vi "System Display Settings.vi"(0 "VISA resource name":refnum<visa-resource-name>, 1 "Result Mode (0:Mode A)":i32(ring) items=["Mode A", "Mode B"], 5 "Enable Sound (1:On)":i32(ring)=1 items=["Off", "On"], 7 "LCD Display Mode (1:On)":i32(ring)=1 items=["Off", "On"], 9 "Uncal Display Mode (1:On)":i32(ring)=1 items=["Off", "On"], 11 "error in (no error)":errorcluster, 12 "Display Title (1:Show Title Display)":i32(ring)=1 items=["No Title Display", "Show Title Display", "Erase Warmup Message"], 13 "Title":string) -> (4 "VISA resource name out":refnum<visa-resource-name>, 15 "error out":errorcluster)   [LabVIEW 2020, in "Anritsu Signal Analyzer Series.lvlib"]
doc: "Sets the system or display settings for sound, LCD, Uncal, and Result mode settings."
uses:
  Anritsu Signal Analyzer Series.lvlib
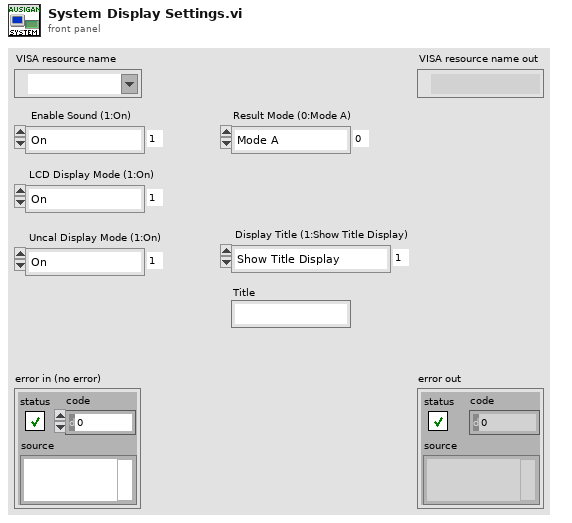
[diagram p1: front panel]
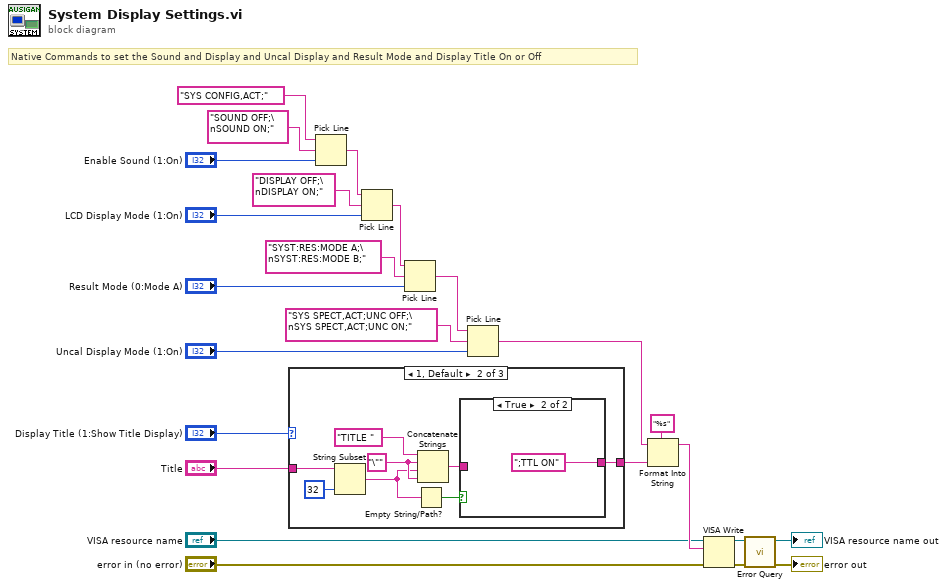
[diagram p0: block diagram]
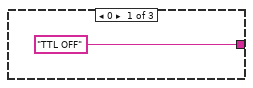
[diagram p2: hidden frame]
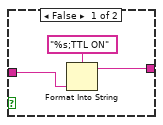
[diagram p3: hidden frame]
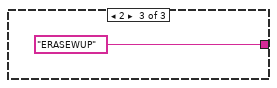
[diagram p4: hidden frame]
diagram:
  # "Native Commands to set the Sound and Display and Uncal Display and Result Mode and Display Title On or Off"
  n1 = case shown="1, Default" "Display Title (1:Show Title Display)" {
    tunnel: ["TTL OFF" ("_CommandSet") w29 "ERASEWUP" ("_CommandSet")] -> w12
    tunnel: "Title" -> [_ w28 _]
    frame 0 {
    }
    frame 1, Default {
      w33 = "\"" ("string")
      n2 = String Subset(string=w28, length (rest)=32 ("length (rest)")) -> (substring=w27:string)  [unwired: 1 in]
      n3 = Empty String/Path?(string/path=w27) -> (empty?=w26:bool)
      n4 = Concatenate Strings("TITLE " ("_CommandSet"), w33, w27, w33) -> (w30:string)
      n5 = case shown="True" w26 {
        tunnel: w30 -> [w35 _]
        tunnel: [w34 ";TTL ON" ("形式文字列")] -> w29
        frame False {
          n6 = Format Into String(format string="%s;TTL ON" ("形式文字列"), w35) -> (resulting string=w34:string)  [unwired: 2 in, 1 out]
        }
        frame True {
        }
      }
    }
    frame 2 {
    }
  }
  n7 = Pick Line(string ("")="SYS CONFIG,ACT;" ("_Case1"), multi-line string="SOUND OFF;\nSOUND ON;" ("_Case1"), line index="Enable Sound (1:On)") -> (output string=w14:string)
  n8 = Pick Line(string ("")=w14, multi-line string="DISPLAY OFF;\nDISPLAY ON;" ("_Case1"), line index="LCD Display Mode (1:On)") -> (output string=w8:string)
  n9 = Pick Line(string ("")=w8, multi-line string="SYST:RES:MODE A;\nSYST:RES:MODE B;" ("_Case1"), line index="Result Mode (0:Mode A)") -> (output string=w1:string)
  n10 = Pick Line(string ("")=w1, multi-line string="SYS SPECT,ACT;UNC OFF;\nSYS SPECT,ACT;UNC ON;" ("_Case1"), line index="Uncal Display Mode (1:On)") -> (output string=w9:string)
  n11 = Format Into String(format string="%s", initial string=w9, w12) -> (resulting string=w7:string)  [unwired: 1 in, 1 out]
  n12 = VISA Write(VISA resource name="VISA resource name", write buffer=w7, error in (no error)="error in (no error)") -> (VISA resource name out=w6:refnum<visa-resource-name>, error out=w5:errorcluster)  [unwired: 1 out]
  n13 = call "Error Query.vi"("error in (no error)"=w5, "VISA resource name"=w6) -> ("error out"=→"error out":errorcluster, "VISA resource name out"=→"VISA resource name out":refnum<visa-resource-name>)  [unwired: 6 in, 2 out]
